vi "JanisDC_4Channel_LKS331_4SRS830.vi"() -> ()   [LabVIEW 2014]
uses:
  <vilib>/Utility/file.llb/Write To Spreadsheet File (DBL).vi
panel:
  out "Probe Temp":dbl format="%.3f"
  out "Cryostat Temp":dbl format="%.3f"
  in  "Tab Control":T1(tab)
  in  "SRS830_4\nAddress":i16
  in  "Start T":dbl=130.0
  in  "T Step":dbl=1.0
  in  "End T":dbl
  in  "Mid T":dbl
  in  "T Step 2":dbl=1.0
  in  "Seconds for Stability":dbl=200.0
  in  "SRS830_1\nAddress":i16
  in  "SRS830_2\nAddress":i16
  in  "Save file path":path
  in  "error in (no error)":errorcluster
  out "error out":errorcluster
  in  "Amplitude":dbl=0.75
  in  "Delay Time (s)":dbl=0.4
  in  "Frequency":dbl=0.1
  in  "Offset":dbl=3.0
  in  "Phase":dbl
  in  "Amplifier Offset":dbl=0.1 caption="Frequency"
  in  "Amplifier Gain":dbl=0.1 caption="Frequency"
  in  "LKS331\nAddress":i16
  in  "Setpoint Proximity":dbl=0.01 format="%#.3g"
  in  "Required Stability":dbl=0.002 format="%#.4g"
  in  "SRS830_3\nAddress":i16
  out "XY Graph 3":cluster{dbl, dbl}[](graph) caption="SRS2"
  out "XY Graph 4":cluster{dbl, dbl}[](graph) caption="SRS1"
  out "XY Graph 5":cluster{dbl, dbl}[](graph) caption="LR700"
  out "XY Graph 6":cluster{dbl, dbl}[](graph) caption="LR700"
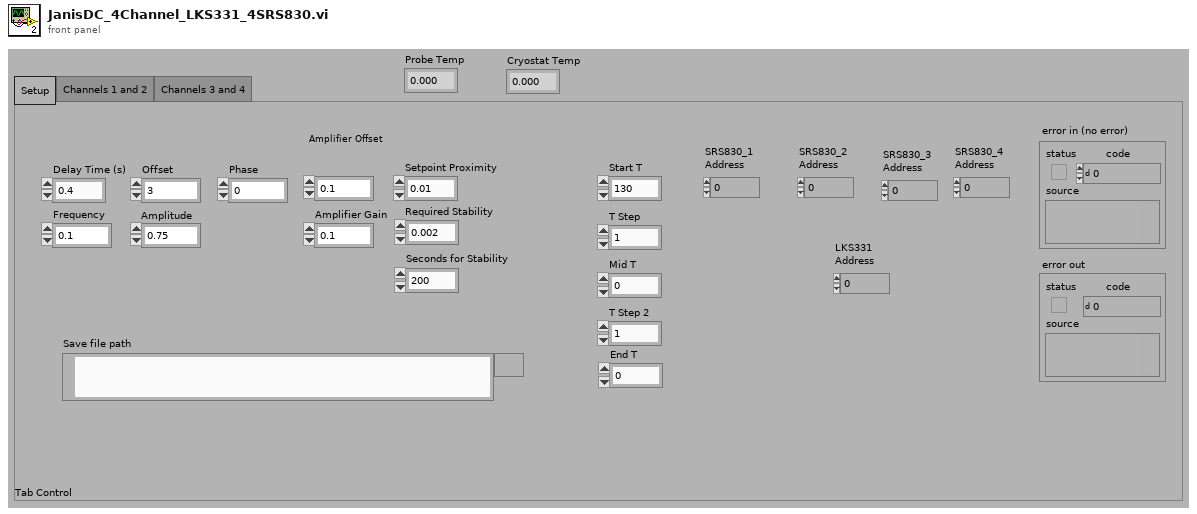
[diagram p1: front panel]
types:
  T1 = enum32{"Setup", "Channels 1 and 2", "Channels 3 and 4"}
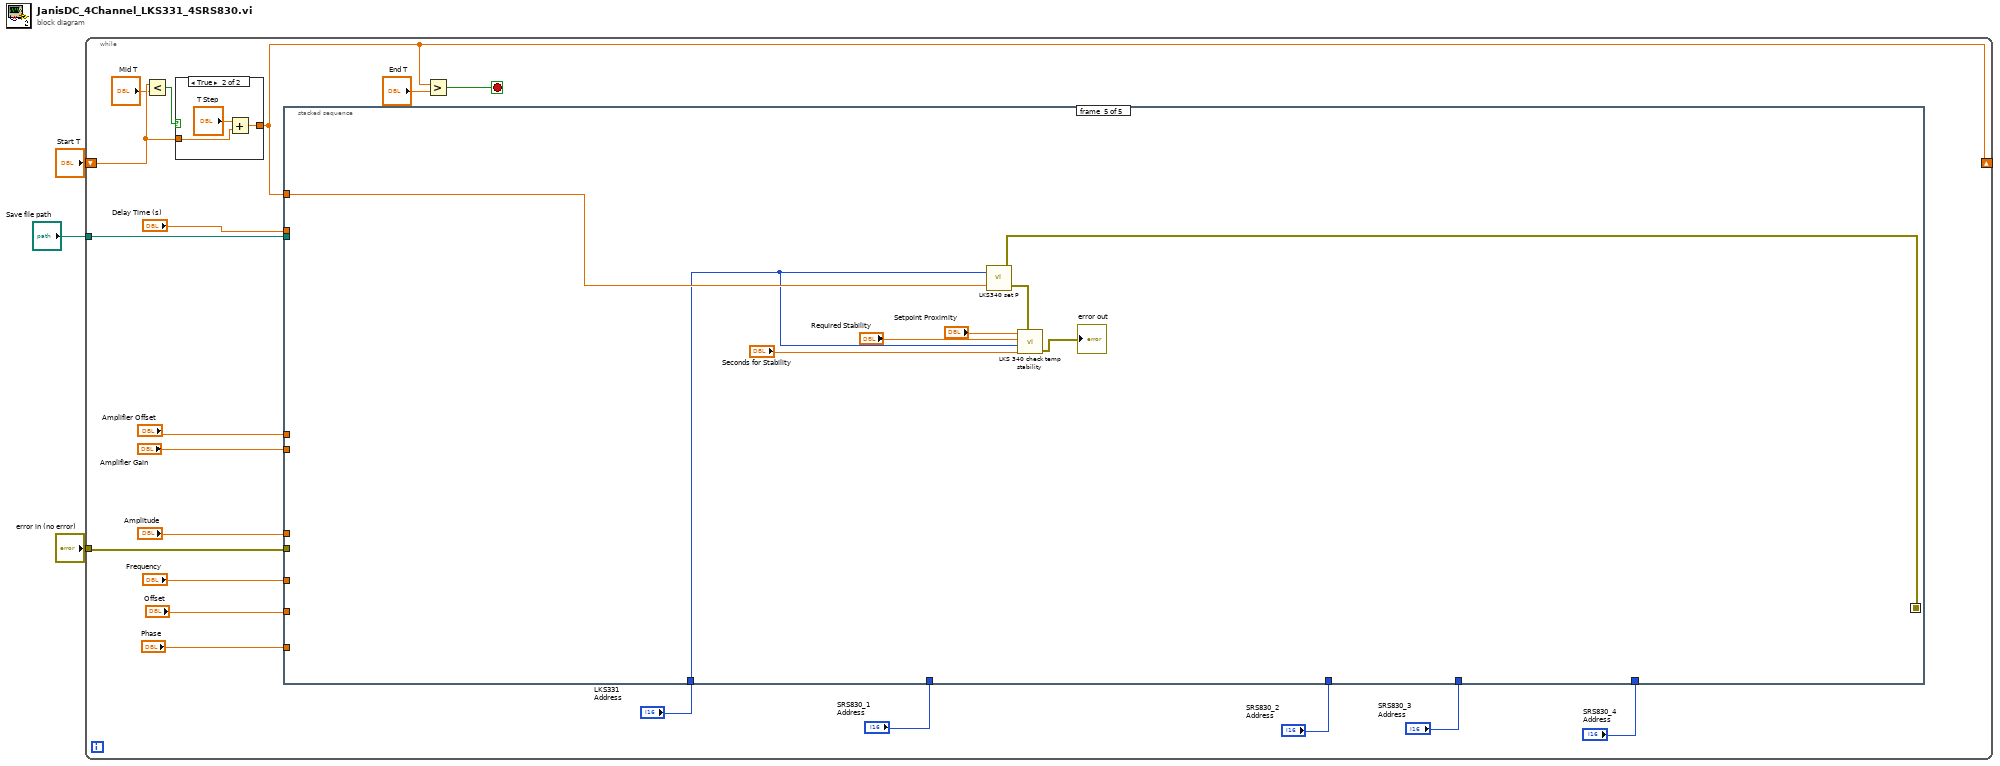
[diagram p0: block diagram]
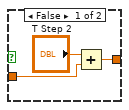
[diagram p2: hidden frame]
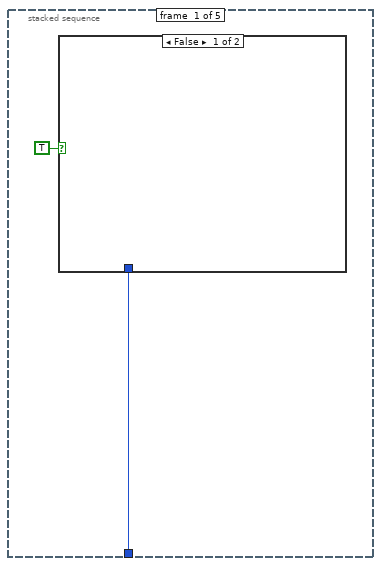
[diagram p3: hidden frame]
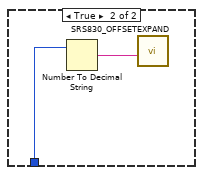
[diagram p4: hidden frame]
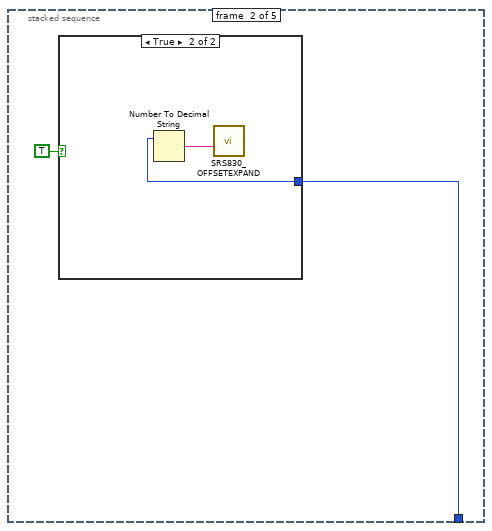
[diagram p5: hidden frame]
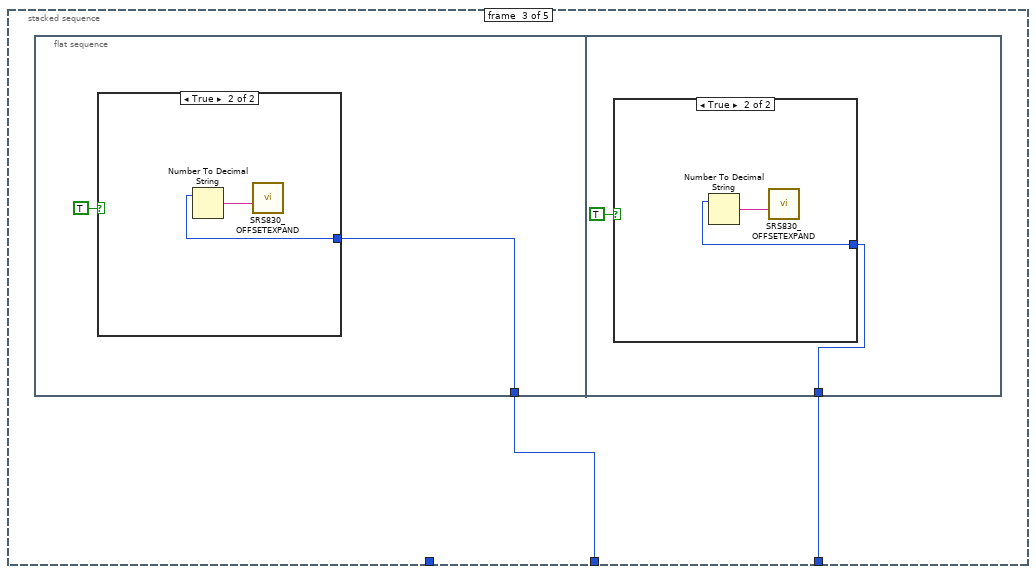
[diagram p7: hidden frame]
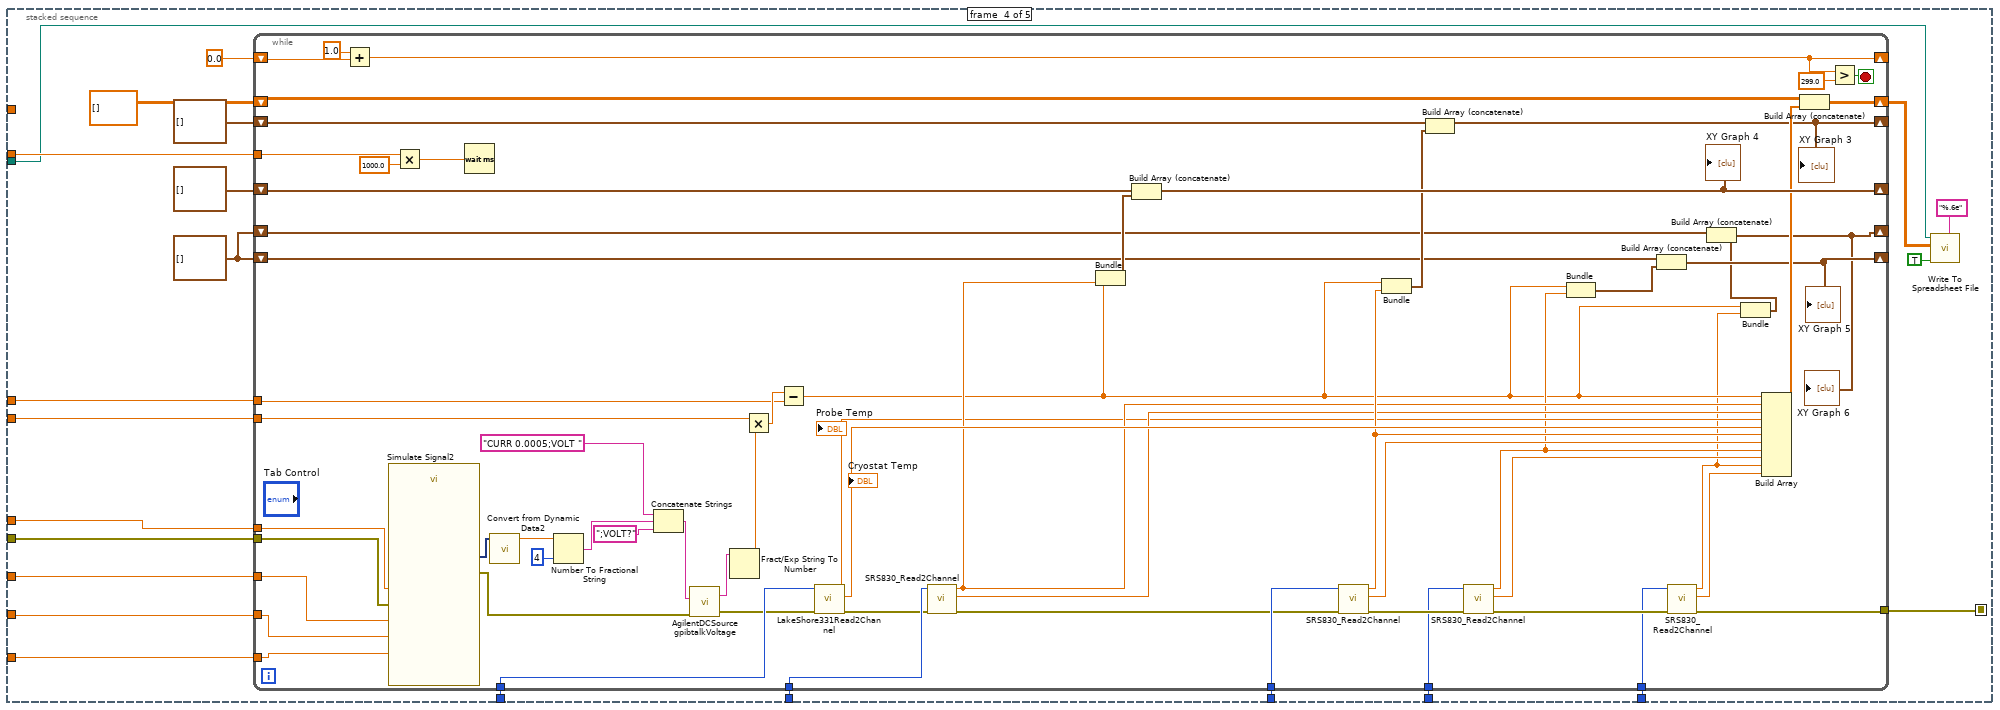
[diagram p10: hidden frame]
diagram:
  n1 = while {
    shift-right: [w18] -> _
    shift-left: "Start T" -> [w21]
    tunnel: "error in (no error)" -> [w17]
    tunnel: "Save file path" -> [w7]
    stop <- w23 stop-if-true
    n2 = Less?(x=w21, y="Mid T") -> (x < y?=w22:bool)
    n3 = case shown="True" w22 {
      tunnel: w21 -> [w25 w28]
      tunnel: [w24 w27] -> w18
      frame False {
        n4 = Add(x="T Step 2", y=w25) -> (x+y=w24:dbl)
      }
      frame True {
        n5 = Add(x="T Step", y=w28) -> (x+y=w27:dbl)
      }
    }
    n6 = stacked-sequence {
      seq-local: [_ _ _ w66 _] -> [_ _ _ _ w134]
      tunnel: w18 -> [_ _ _ _ w141]
      tunnel: w17 -> [_ _ _ w67 _]
      tunnel: "SRS830_1\nAddress" -> [w31 _ _ w64 _]
      tunnel: "SRS830_2\nAddress" -> [_ w35 _ w63 _]
      tunnel: "Amplitude" -> [_ _ _ w62 _]
      tunnel: "Frequency" -> [_ _ _ w61 _]
      tunnel: "Offset" -> [_ _ _ w60 _]
      tunnel: "Phase" -> [_ _ _ w59 _]
      tunnel: "Delay Time (s)" -> [_ _ _ w58 _]
      tunnel: "Amplifier Gain" -> [_ _ _ w57 _]
      tunnel: "Amplifier Offset" -> [_ _ _ w56 _]
      tunnel: w7 -> [_ _ _ w52 _]
      tunnel: "LKS331\nAddress" -> [_ _ _ w51 w135]
      tunnel: "SRS830_3\nAddress" -> [_ _ w39 w50 _]
      tunnel: "SRS830_4\nAddress" -> [_ _ w38 w48 _]
      frame #0 {
        n7 = case shown="False" TRUE {
          tunnel: w31 -> [_ w32]
          frame False {
          }
          frame True {
            n8 = Number To Decimal String(number=w32) -> (decimal integer string=w33:string)  [unwired: 1 in]
            n9 = call "SRS830_OFFSETEXPAND.vi"("address string"=w33) -> ()  [unwired: 11 in]
          }
        }
      }
      frame #1 {
        n10 = case shown="True" TRUE {
          tunnel: w35 -> [_ w36]
          frame False {
          }
          frame True {
            n11 = Number To Decimal String(number=w36) -> (decimal integer string=w37:string)  [unwired: 1 in]
            n12 = call "SRS830_OFFSETEXPAND.vi"("address string"=w37) -> ()  [unwired: 11 in]
          }
        }
      }
      frame #2 {
        n13 = flat-sequence {
          tunnel: w39 -> [w40]
          tunnel: w38 -> [w44]
          frame #0 {
            n14 = case shown="True" TRUE {
              tunnel: w40 -> [_ w42]
              frame False {
              }
              frame True {
                n15 = Number To Decimal String(number=w42) -> (decimal integer string=w43:string)  [unwired: 1 in]
                n16 = call "SRS830_OFFSETEXPAND.vi"("address string"=w43) -> ()  [unwired: 11 in]
              }
            }
          }
          frame #1 {
            n17 = case shown="True" TRUE {
              tunnel: w44 -> [_ w46]
              frame False {
              }
              frame True {
                n18 = Number To Decimal String(number=w46) -> (decimal integer string=w47:string)  [unwired: 1 in]
                n19 = call "SRS830_OFFSETEXPAND.vi"("address string"=w47) -> ()  [unwired: 11 in]
              }
            }
          }
        }
      }
      frame #3 {
        w49 = cluster{dbl, dbl}[] []
        n20 = while {
          shift-right: [w126] -> _
          shift-left: cluster{dbl, dbl}[] [] -> [w112]
          shift-right: [w124] -> w53
          shift-left: dbl[][] [] -> [w125]
          shift-right: [w120] -> _
          shift-left: 0.0 -> [w123]
          tunnel: w67 -> [w115]
          tunnel: [w78] -> w66
          shift-right: [w100] -> _
          shift-left: cluster{dbl, dbl}[] [] -> [w110]
          tunnel: w64 -> [w97]
          tunnel: w63 -> [w96]
          tunnel: w62 -> [w107]
          tunnel: w61 -> [w106]
          tunnel: w60 -> [w105]
          tunnel: w59 -> [w104]
          tunnel: w58 -> [w103]
          tunnel: w57 -> [w102]
          tunnel: w56 -> [w89]
          tunnel: w51 -> [w99]
          shift-right: [w87] -> _
          shift-left: w49 -> [w86]
          tunnel: w50 -> [w82]
          shift-right: [w71] -> _
          shift-left: w49 -> [w74]
          tunnel: w48 -> [w77]
          stop <- w121 stop-if-true
          n21 = Add(x=1.0, y=w123) -> (x+y=w120:dbl)
          n22 = call "Simulate Signal2"("Offset"=w105, "Frequency"=w106, "Amplitude"=w107, "Phase"=w104, "error in (no error)"=w115) -> ("Triangle"=w133:dynamicdata, "error out"=w114:errorcluster)  [unwired: 9 in]
          n23 = Multiply(x=w103, y=1000.0) -> (x*y=w117:dbl)
          n24 = Wait (ms)(milliseconds to wait=w117) -> ()  [unwired: 1 out]
          n25 = call "Convert from Dynamic Data2"("Dynamic Data Type"=w133) -> ("Scalar"=w132:dbl)  [unwired: 3 in]
          n26 = Number To Fractional String(number=w132, precision (6)=4) -> (F-format string=w131:string)  [unwired: 2 in]
          n27 = Concatenate Strings("CURR 0.0005;VOLT ", w131, ";VOLT?") -> (w127:string)
          n28 = call "AgilentDCSource gpibtalkVoltage.vi"("error in"=w114, "Send"=w127) -> ("error out"=w98:errorcluster, "read"=w108:string)  [unwired: 2 in]
          n29 = Fract/Exp String To Number(string=w108) -> (number=w109:dbl)  [unwired: 3 in, 1 out]
          n30 = Multiply(x=w102, y=w109) -> (x*y=w116:dbl)
          n31 = Subtract(x=w116, y=w89) -> (x-y=w75:dbl)
          n32 = call "LakeShore331Read2Channel.vi"("error in (no error)"=w98, "LKS331\nGPIB Address"=w99) -> ("error out"=w95:errorcluster, "TempCryostat"=w93:dbl, "TempProbe"=w84:dbl)  [unwired: 7 in]
          "Cryostat Temp" <- w93
          "Probe Temp" <- w84
          n33 = call "SRS830_Read2Channel.vi"("error in (no error)"=w95, "Lock in\nGPIB Address"=w97) -> ("error out"=w94:errorcluster, "Ch_OUTP3"=w88:dbl, "Ch_OUTR1"=w90:dbl)  [unwired: 7 in]
          n34 = Bundle(w75, "Ch_OUTR1"=w90) -> (w111:cluster{dbl, "Ch_OUTR1":dbl})  [unwired: 1 in]
          n35 = Build Array (concatenate)(w112, w111) -> (w126:cluster{dbl, "Ch_OUTR1":dbl}[])
          "XY Graph 4" <- w126
          n36 = call "SRS830_Read2Channel.vi"("error in (no error)"=w94, "Lock in\nGPIB Address"=w96) -> ("error out"=w83:errorcluster, "Ch_OUTP3"=w91:dbl, "Ch_OUTR1"=w92:dbl)  [unwired: 7 in]
          n37 = Bundle(w75, "Ch_OUTR1"=w92) -> (w113:cluster{dbl, "Ch_OUTR1":dbl})  [unwired: 1 in]
          n38 = Build Array (concatenate)(w110, w113) -> (w100:cluster{dbl, "Ch_OUTR1":dbl}[])
          "XY Graph 3" <- w100
          n39 = call "SRS830_Read2Channel.vi"("error in (no error)"=w83, "Lock in\nGPIB Address"=w82) -> ("error out"=w79:errorcluster, "Ch_OUTP3"=w81:dbl, "Ch_OUTR1"=w80:dbl)  [unwired: 7 in]
          n40 = Bundle(w75, "Ch_OUTR1"=w80) -> (w85:cluster{dbl, "Ch_OUTR1":dbl})  [unwired: 1 in]
          n41 = Build Array (concatenate)(w86, w85) -> (w87:cluster{dbl, "Ch_OUTR1":dbl}[])
          "XY Graph 5" <- w87
          n42 = call "SRS830_Read2Channel.vi"("error in (no error)"=w79, "Lock in\nGPIB Address"=w77) -> ("error out"=w78:errorcluster, "Ch_OUTP3"=w76:dbl, "Ch_OUTR1"=w73:dbl)  [unwired: 7 in]
          n43 = Bundle(w75, "Ch_OUTR1"=w73) -> (w72:cluster{dbl, "Ch_OUTR1":dbl})  [unwired: 1 in]
          n44 = Build Array (concatenate)(w74, w72) -> (w71:cluster{dbl, "Ch_OUTR1":dbl}[])
          "XY Graph 6" <- w71
          n45 = Build Array(w75, w90, w88, w84, w93, w92, w91, w80, w81, w73, w76) -> (w101:dbl[])
          n46 = Build Array (concatenate)(w125, w101) -> (w124:dbl[][])
          n47 = Greater?(x=w120, y=299.0) -> (0:w121:bool)
        }
        n48 = call-poly <vilib>:"Write To Spreadsheet File.vi"("format (%.3f)"="%.6e", "append to file? (new file:F)"=TRUE, "2D data"=w53, "file path (dialog if empty)"=w52) -> ()  [unwired: 4 in, 1 out]
      }
      frame #4 {
        n49 = call "LKS340 set P.vi"("error in"=w134, "Set point"=w141, "GPIB Adress"=w135) -> ("error out"=w139:errorcluster)
        n50 = call "LKS 340 check temp stability.vi"("Set point proximity"="Setpoint Proximity", "Stability"="Required Stability", "GPIB Address"=w135, "seconds to wait"="Seconds for Stability", "error in"=w139) -> ("error out"=→"error out":errorcluster)  [unwired: 2 in]
      }
    }
    n51 = Greater?(x=w18, y="End T") -> (0:w23:bool)
  }
